vi "240126_String2Axis.vi"(8 "error in (no error)":errorcluster, 11 "String":string) -> (0 "error out":errorcluster, 1 "++ ou --":bool, 2 "Index":i32, 3 "+-":bool)   [LabVIEW 2023]
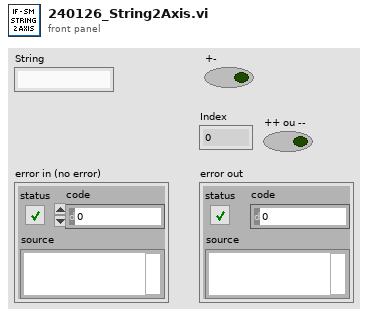
[diagram p1: front panel]
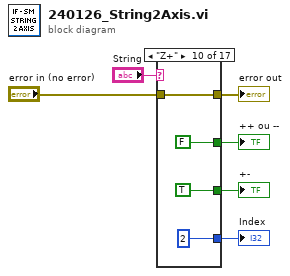
[diagram p0: block diagram]
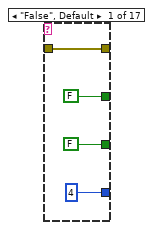
[diagram p2: hidden frame]
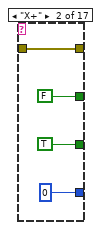
[diagram p3: hidden frame]
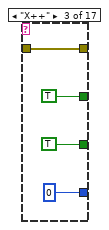
[diagram p4: hidden frame]
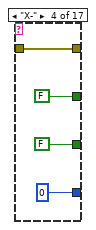
[diagram p5: hidden frame]
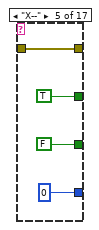
[diagram p6: hidden frame]
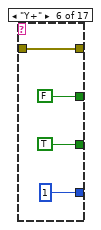
[diagram p7: hidden frame]
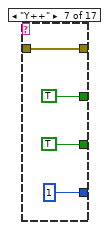
[diagram p8: hidden frame]
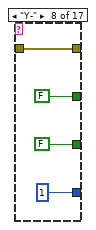
[diagram p9: hidden frame]
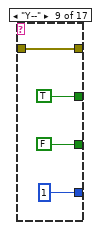
[diagram p10: hidden frame]
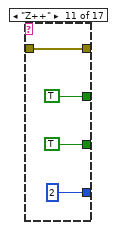
[diagram p11: hidden frame]
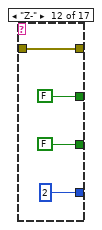
[diagram p12: hidden frame]
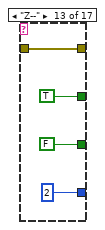
[diagram p13: hidden frame]
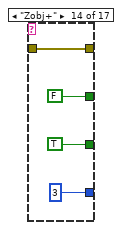
[diagram p14: hidden frame]
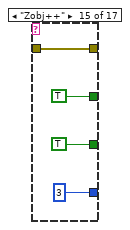
[diagram p15: hidden frame]
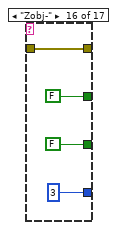
[diagram p16: hidden frame]
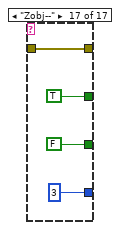
[diagram p17: hidden frame]
diagram:
  n1 = case shown="\"Z+\"" "String" {
    tunnel: "error in (no error)" -> [w10 w14 w16 w22 w26 w30 w34 w38 w42 w46 w48 w54 w58 w62 w66 w70 w72]
    tunnel: [w10 w14 w16 w22 w26 w30 w34 w38 w42 w46 w48 w54 w58 w62 w66 w70 w72] -> w4
    tunnel: [FALSE TRUE TRUE FALSE FALSE TRUE TRUE FALSE FALSE TRUE TRUE FALSE FALSE TRUE TRUE FALSE FALSE] -> w5
    tunnel: [4 0 0 0 0 1 1 1 1 2 2 2 2 3 3 3 3] -> w6
    tunnel: [FALSE ("++ ou --") FALSE ("++ ou --") TRUE ("++ ou --") FALSE ("++ ou --") TRUE ("++ ou --") FALSE ("++ ou --") TRUE ("++ ou --") FALSE ("++ ou --") TRUE ("++ ou --") FALSE ("++ ou --") TRUE ("++ ou --") FALSE ("++ ou --") TRUE ("++ ou --") FALSE ("++ ou --") TRUE ("++ ou --") FALSE ("++ ou --") TRUE ("++ ou --")] -> w1
    frame "False", Default {
    }
    frame "X+" {
    }
    frame "X++" {
    }
    frame "X-" {
    }
    frame "X--" {
    }
    frame "Y+" {
    }
    frame "Y++" {
    }
    frame "Y-" {
    }
    frame "Y--" {
    }
    frame "Z+" {
    }
    frame "Z++" {
    }
    frame "Z-" {
    }
    frame "Z--" {
    }
    frame "Zobj+" {
    }
    frame "Zobj++" {
    }
    frame "Zobj-" {
    }
    frame "Zobj--" {
    }
  }
  "Index" <- w6
  "+-" <- w5
  "error out" <- w4
  "++ ou --" <- w1
